vi "Panel.vi"(11 "GettingStarted in":refnum<class "GettingStarted.lvclass">) -> ()   [LabVIEW 2020, in "PicoG-App.lvlib" / "GettingStarted.lvclass"]
uses:
  GettingStarted.lvclass
  <vilib>/IlluminatedG/IG OOPanel/OOPanel/Panel/Panel.lvclass
  <vilib>/IlluminatedG/IG OOPanel/OOPanel/OOPanel.lvlib
  C:/Program Files (x86)/National Instruments/LabVIEW 2020/vi.lib/IlluminatedG/IG OOPanel/OOPanel/Panel/Panel.lvclass
  C:/dev/Vireo/PicoG/PicoG-App/GettingStarted/GettingStarted.lvclass
panel:
  in  "Nav Platforms":bool
  # "It looks like you don't have any devices or applications set up yet!\n\nClick below to get started with setting up your first device and running your first application:"
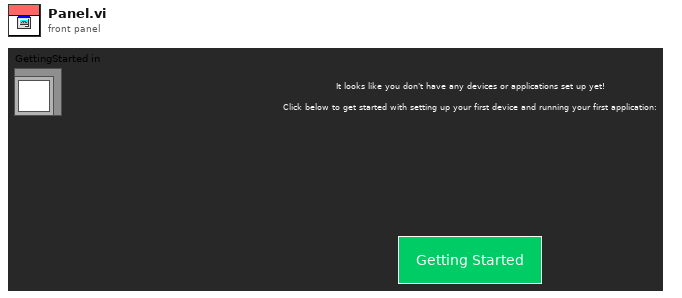
[diagram p1: front panel]
types:
  T1 = typedef "OOPanel.lvlib/Panel.lvclass/Panel Events.ctl" = cluster{"Visbility":refnum<user-event>, "Close":refnum<user-event>}
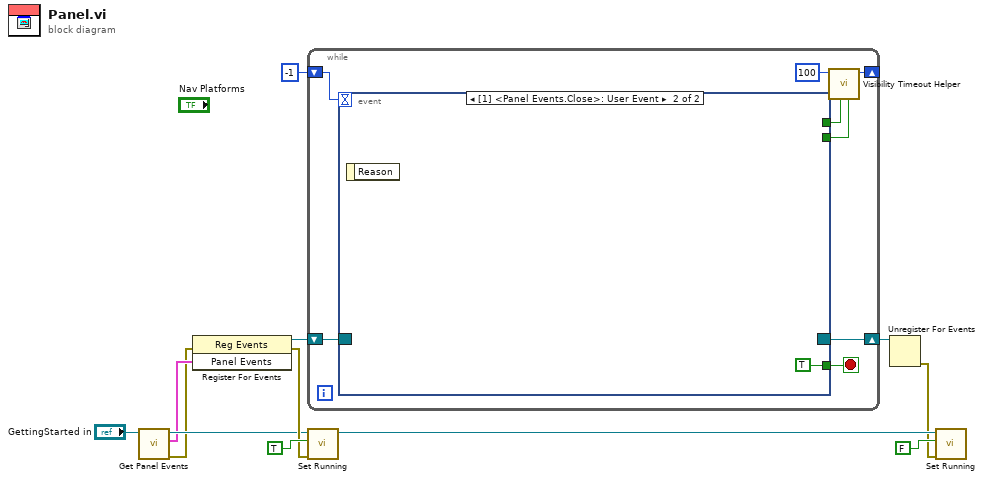
[diagram p0: block diagram]
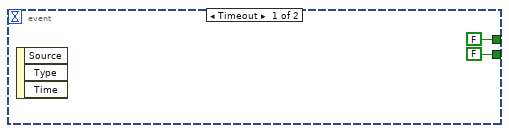
[diagram p2: hidden frame]
diagram:
  n1 = call <vilib>:"Get Panel Events.vi"("Panel in"="GettingStarted in") -> ("error out"=w3:errorcluster, "Panel Events"=w4:T1, "Panel out"=w5:refnum<class "GettingStarted.lvclass">)  [unwired: 8 in]
  n2 = register-events(error in=w3, w4) -> (reference out=w9:refnum<event-registration>, error out=w6:errorcluster)  [unwired: 1 in]
  n3 = while {
    shift-right: [w16] -> w11
    shift-left: w9 -> [w17]
    shift-right: [w19] -> _
    shift-left: -1 ("Timeout") -> [w18]
    stop <- w13 stop-if-true
    n4 = event shown="[1] <Panel Events.Close>: User Event" {
      selector: w17 -> [_ _]
      dyn-events: [_ _] -> w16
      timeout: w18 -> [_ _]
      tunnel: [FALSE _] -> w15
      tunnel: [FALSE _] -> w14
      tunnel: [_ TRUE] -> w13
      event Timeout {
        n5 = event-data() -> ()  [unwired: 1 in, 3 out]
      }
      event User Event {
        n6 = event-data() -> ()  [unwired: 1 in, 1 out]
      }
    }
    n7 = call <vilib>:"Visibility Timeout Helper.vi"("Update?"=w14, "Use Timeout?"=w15, "Visible Timeout mS"=100) -> ("Timeout"=w19:i32)  [unwired: 8 in]
  }
  n8 = call <vilib>:"Set Running.vi"("error in (no error)"=w6, "Running"=TRUE, "Panel in"=w5) -> ("Panel out"=w12:refnum<class "GettingStarted.lvclass">)  [unwired: 7 in, 1 out]
  n9 = Unregister For Events(event registration refnum=w11) -> (error out=w2:errorcluster)  [unwired: 1 in]
  n10 = call <vilib>:"Set Running.vi"("error in (no error)"=w2, "Running"=FALSE, "Panel in"=w12) -> ()  [unwired: 7 in, 2 out]
